vi "Read 1Chan 1Samp 1D SGL.vi"(8 "error in (no error)":errorcluster, 11 "MicroDAQ.lvlib:Analog Input.lvclass":refnum<class "Analog Input.lvclass">) -> (0 "error out":errorcluster, 2 "Value":dbl, 3 "MicroDAQ.lvlib:Analog Input.lvclass out":refnum<class "Analog Input.lvclass">)   [LabVIEW 2009, in "MicroDAQ.lvlib" / "Analog Input.lvclass"]
doc: "Reads a single floating-point sample from a channel."
uses:
  <instrlib>/MicroDAQ/Channel/Analog Input/Analog Input.lvclass
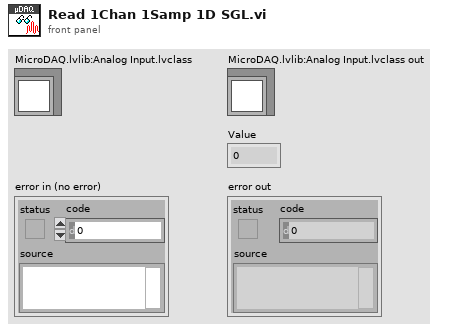
[diagram p1: front panel]
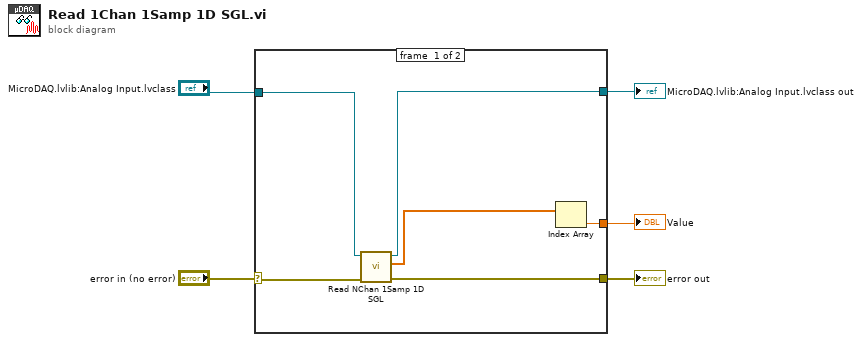
[diagram p0: block diagram]
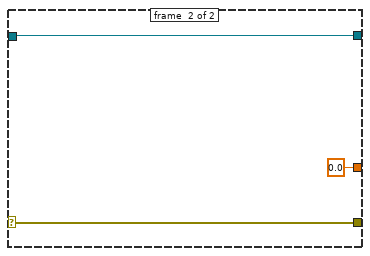
[diagram p2: hidden frame]
diagram:
  n1 = case shown="No Error" "error in (no error)" {
    selector: "error in (no error)" -> [w11 w13]
    tunnel: [w6 w13] -> w4
    tunnel: [w7 w14] -> w3
    tunnel: "MicroDAQ.lvlib:Analog Input.lvclass" -> [w10 w14]
    tunnel: [w9 0.0] -> w1
    frame #0 {
      n2 = call <instrlib>:"Read NChan 1Samp 1D SGL.vi"("error in (no error)"=w11, "MicroDAQ.lvlib:Analog Input.lvclass"=w10) -> ("error out"=w6:errorcluster, "Values"=w8:dbl[], "MicroDAQ.lvlib:Analog Input.lvclass out"=w7:refnum<class "Analog Input.lvclass">)  [unwired: 7 in]
      n3 = Index Array(array=w8) -> (element=w9:dbl)  [unwired: 1 in]
    }
    frame #1 {
    }
  }
  "error out" <- w4
  "MicroDAQ.lvlib:Analog Input.lvclass out" <- w3
  "Value" <- w1
